vi "KB-ShowBasePoint.vi"(8 "error in (no error)":errorcluster, 10 "Create Flatnesss Base Point":cluster{"X":dbl, "Y":dbl, "Z":dbl}[](array[cluster]), 11 "Image In":T1(plugin-control)) -> (0 "error out":errorcluster, 3 "Image Out":T1(plugin-control))   [LabVIEW 2015]
panel:
  out "数值":i32
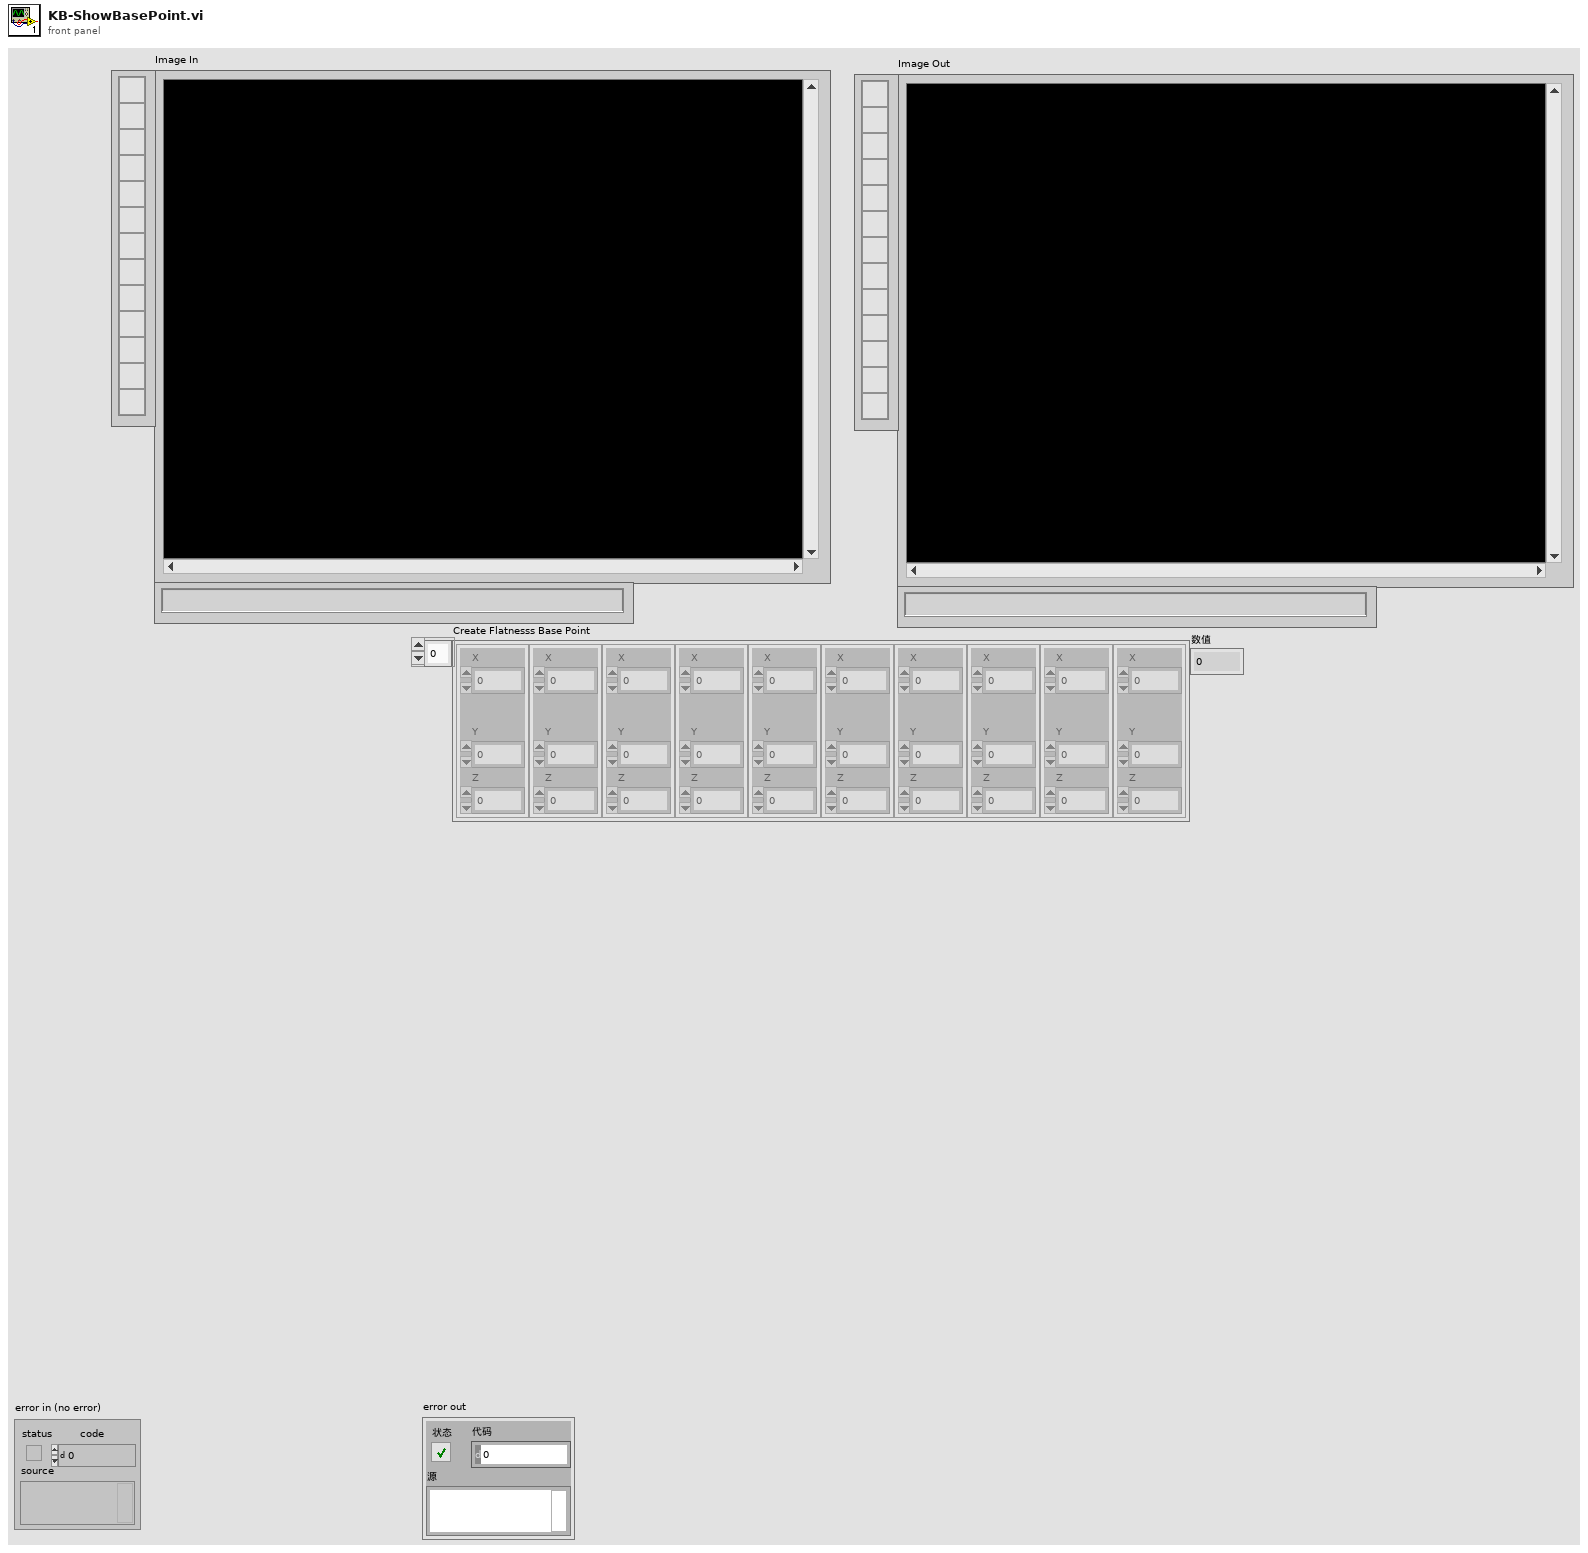
[diagram p1: front panel]
types:
  T1 = typedef "IMAQ Image.ctl" = refnum<image>
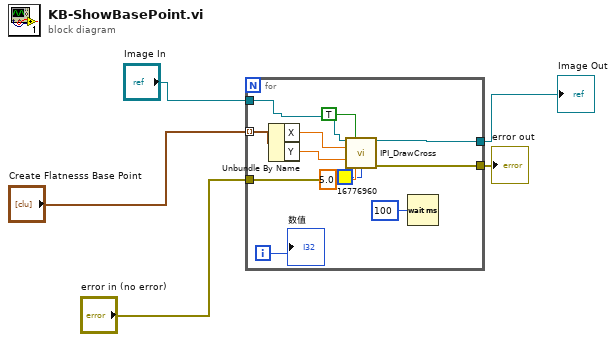
[diagram p0: block diagram]
diagram:
  n1 = for {
    tunnel: "Create Flatnesss Base Point" -> [w17] mode=indexing
    tunnel: [w9] -> w1
    tunnel: "error in (no error)" -> [w12]
    tunnel: [w11] -> w3
    tunnel: "Image In" -> [w10]
    i -> [w8]
    n2 = Unbundle By Name(w17) -> ("X"=w16:dbl, "Y"=w15:dbl)
    n3 = call "IPI_DrawCross.vi"("Image In"=w10, "Show Cross"=TRUE, "X"=w16, "Y"=w15, "error in (no error)"=w12, "Radius"=5.0, "颜色盒"=u32 16776960) -> ("Image Out"=w9:T1, "error out"=w11:errorcluster)  [unwired: 7 in]
    n4 = Wait (ms)(milliseconds to wait=u32 100 ("等待时间（毫秒）")) -> ()  [unwired: 1 out]
    "数值" <- w8
  }
  "error out" <- w3
  "Image Out" <- w1
